vi "DAC Configure.vi"(8 "error in":errorcluster, 11 "DAC HeatFlow AIV in":refnum<class "DAC HeatFlow AOV.lvclass">) -> (0 "error out":errorcluster, 3 "DAC HeatFlow AIV out":refnum<class "DAC HeatFlow AOV.lvclass">)   [LabVIEW 2019, in "DAC.lvlib" / "DAC HeatFlow AOV.lvclass"]
uses:
  DAC HeatFlow AOV.lvclass
  C:/Users/krio/Documents/LV_Projects/test-stand/App/DAC/DAC.lvclass
  DAC.lvclass/DAC.ctl
  DAC HeatFlow AOV.lvclass/DAC HeatFlow AOV.ctl
  <vilib>/Utility/error.llb/Error Cluster From Error Code.vi
  <vilib>/DAQmx/create/channels.llb/DAQmx Create Channel (AI-Voltage-Basic).vi
  <vilib>/DAQmx/configure/timing.llb/DAQmx Timing (Sample Clock).vi
  <vilib>/ErrorRing/Error Ring.xnode
  DAC.lvclass
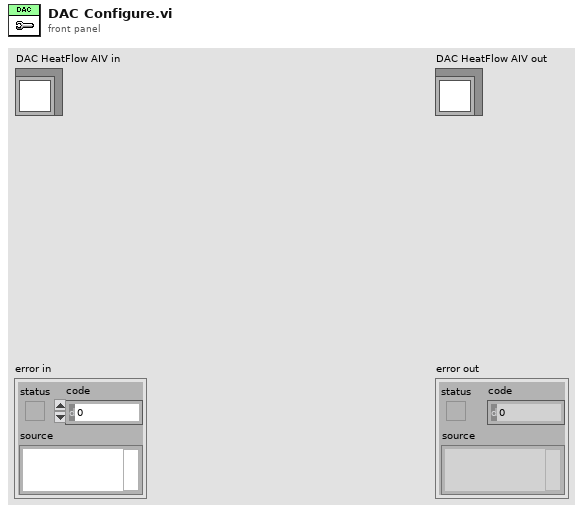
[diagram p1: front panel]
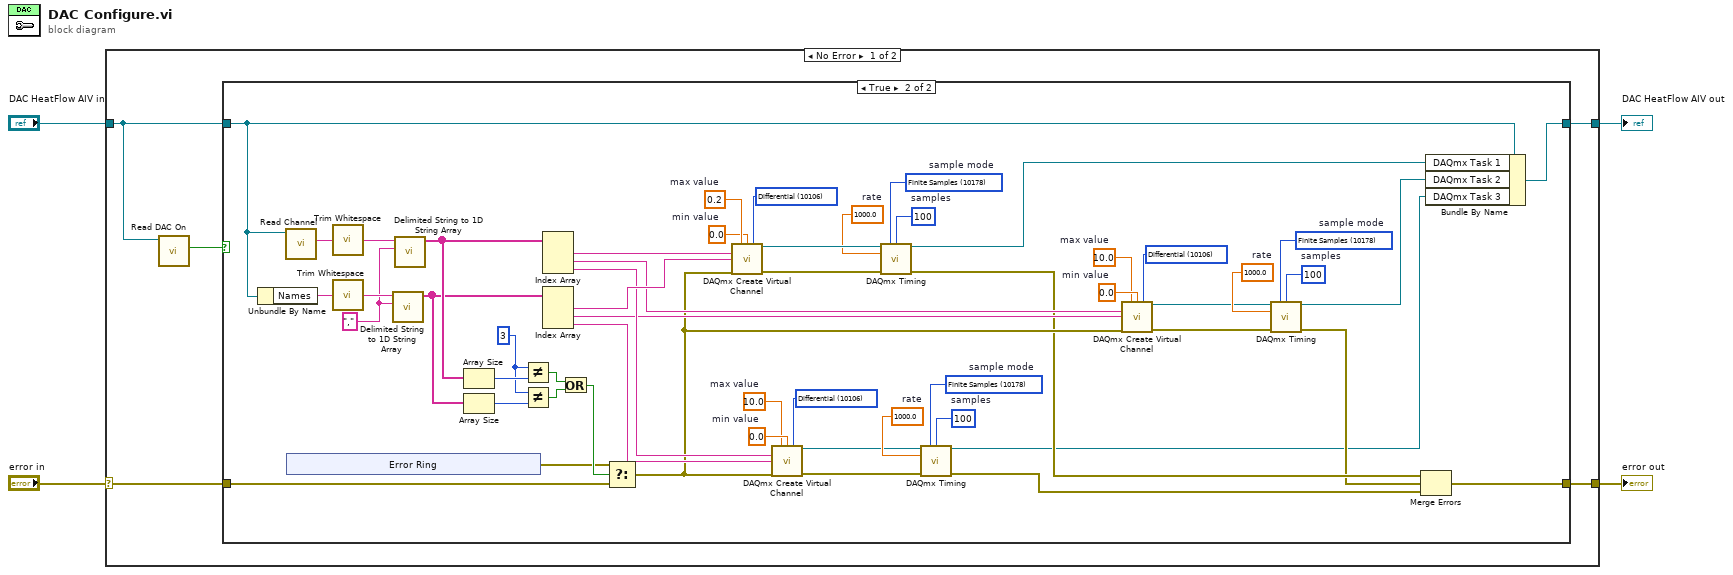
[diagram p0: block diagram]
diagram:
  n1 = case shown="No Error" "error in" {
    selector: "error in" -> [w6 w72]
    tunnel: [w5 w72] -> w4
    tunnel: [w7 w71] -> w3
    tunnel: "DAC HeatFlow AIV in" -> [w9 w71]
    frame No Error {
      n2 = call "Read DAC On.vi"("DAC in"=w9) -> ("DAC On"=w8:bool)  [unwired: 8 in, 2 out]
      n3 = case shown="True" w8 {
        tunnel: w9 -> [w11 w65]
        tunnel: [w11 w66] -> w7
        tunnel: w6 -> [w10 w44]
        tunnel: [w10 w14] -> w5
        frame False {
        }
        frame True {
          w30 = 10106 items=["Default"=-1, "RSE"=10083, "NRSE"=10078, "Differential"=10106, "Pseudodifferential"=12529] ("input terminal configuration")
          w29 = 0.0  # min value
          w28 = 10.0  # max value
          w27 = 100  # samples
          w26 = 1000.0  # rate
          w25 = 10178 items=["Finite Samples"=10178, "Continuous Samples"=10123, "Hardware Timed Single Point"=12522]  # sample mode
          w38 = 10106 items=["Default"=-1, "RSE"=10083, "NRSE"=10078, "Differential"=10106, "Pseudodifferential"=12529] ("input terminal configuration")
          w37 = 0.0  # min value
          w36 = 10.0  # max value
          w35 = 100  # samples
          w34 = 1000.0  # rate
          w33 = 10178 items=["Finite Samples"=10178, "Continuous Samples"=10123, "Hardware Timed Single Point"=12522]  # sample mode
          w48 = 3 ("x")
          w51 = "," ("delimiter")
          w57 = 10106 items=["Default"=-1, "RSE"=10083, "NRSE"=10078, "Differential"=10106, "Pseudodifferential"=12529] ("input terminal configuration")
          w58 = 0.0  # min value
          w59 = 0.2  # max value
          w60 = 100  # samples
          w61 = 1000.0  # rate
          w62 = 10178 items=["Finite Samples"=10178, "Continuous Samples"=10123, "Hardware Timed Single Point"=12522]  # sample mode
          n4 = Unbundle By Name(w65) -> ("Names"=w54:string)
          n5 = call "Read Channel.vi"("DAC in"=w65) -> ("Channel"=w55:string)  [unwired: 8 in, 2 out]
          n6 = xnode "Error Ring"() -> ("error out"=w43:errorcluster)
          n7 = call <vilib>:"Trim Whitespace.vi"("string"=w55) -> ("trimmed string"=w53:string)  [unwired: 1 in]
          n8 = call <vilib>:"Trim Whitespace.vi"("string"=w54) -> ("trimmed string"=w52:string)  [unwired: 1 in]
          n9 = call <vilib>:"Delimited String to 1D String Array.vi"("delimiter"=w51, "delimited string"=w52) -> ("string array"=w41:string[])  [unwired: 9 in]
          n10 = call <vilib>:"Delimited String to 1D String Array.vi"("delimiter"=w51, "delimited string"=w53) -> ("string array"=w42:string[])  [unwired: 9 in]
          n11 = Array Size(array=w42) -> (size(s)=w50:i32)
          n12 = Array Size(array=w41) -> (size(s)=w49:i32)
          n13 = Not Equal?(x=w48, y=w50) -> (x != y?=w47:bool)
          n14 = Not Equal?(x=w48, y=w49) -> (x != y?=w46:bool)
          n15 = Index Array(array=w42) -> (element #1=w40:string, element #2=w22:string, element #3=w21:string)  [unwired: 3 in]
          n16 = Index Array(array=w41) -> (element #1=w39:string, element #2=w20:string, element #3=w19:string)  [unwired: 3 in]
          n17 = Or(x=w47, y=w46) -> (x .or. y?=w45:bool)
          n18 = Select(t=w43, s=w45, f=w44) -> (s? t:f=w18:errorcluster)
          n19 = call-poly <vilib>:"DAQmx Create Virtual Channel.vi"("maximum value"=w59, "minimum value"=w58, "input terminal configuration"=w57, "physical channels"=w40, "name to assign"=w39, "error in"=w18) -> ("task out"=w64:refnum<k21>, "error out"=w63:errorcluster)  [unwired: 8 in]
          n20 = call-poly <vilib>:"DAQmx Create Virtual Channel.vi"("maximum value"=w28, "minimum value"=w29, "input terminal configuration"=w30, "physical channels"=w21, "name to assign"=w19, "error in"=w18) -> ("task out"=w23:refnum<k21>, "error out"=w24:errorcluster)  [unwired: 8 in]
          n21 = call-poly <vilib>:"DAQmx Timing.vi"("task/channels in"=w64, "sample mode"=w62, "samples per channel"=w60, "rate"=w61, "error in"=w63) -> ("task out"=w56:refnum<k21>, "error out"=w17:errorcluster)  [unwired: 9 in]
          n22 = call-poly <vilib>:"DAQmx Timing.vi"("task/channels in"=w23, "sample mode"=w25, "samples per channel"=w27, "rate"=w26, "error in"=w24) -> ("task out"=w12:refnum<k21>, "error out"=w15:errorcluster)  [unwired: 9 in]
          n23 = call-poly <vilib>:"DAQmx Create Virtual Channel.vi"("maximum value"=w36, "minimum value"=w37, "input terminal configuration"=w38, "physical channels"=w22, "name to assign"=w20, "error in"=w18) -> ("task out"=w31:refnum<k21>, "error out"=w32:errorcluster)  [unwired: 8 in]
          n24 = call-poly <vilib>:"DAQmx Timing.vi"("task/channels in"=w31, "sample mode"=w33, "samples per channel"=w35, "rate"=w34, "error in"=w32) -> ("task out"=w13:refnum<k21>, "error out"=w16:errorcluster)  [unwired: 9 in]
          n25 = Merge Errors(w17, w16, w15) -> (w14:errorcluster)
          n26 = Bundle By Name(cluster=w65, "DAQmx Task 1"=w56, "DAQmx Task 2"=w13, "DAQmx Task 3"=w12) -> (w66:refnum<class "DAC HeatFlow AOV.lvclass">)
        }
      }
    }
    frame Error {
    }
  }
  "error out" <- w4
  "DAC HeatFlow AIV out" <- w3
